vi "Set Configurations.vi"(10 "Configurations":refnum<class "Component Configurations.lvclass">, 11 "Component in":refnum<class "Component.lvclass">) -> (3 "Component out":refnum<class "Component.lvclass">)   [LabVIEW 2019, in "DSF Core.lvlib" / "Component.lvclass"]
uses:
  Component.lvclass
  Component Configuration/Component Configurations.lvclass
  Component.lvclass/Component.ctl
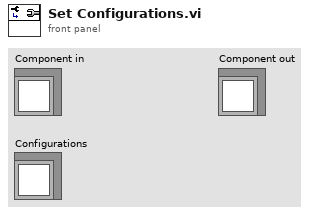
[diagram p1: front panel]
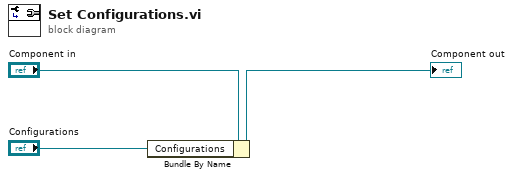
[diagram p0: block diagram]
diagram:
  n1 = Bundle By Name(cluster="Component in", "Configurations"="Configurations") -> (→"Component out":refnum<class "Component.lvclass">)
